vi "Create File.vi"(8 "error in (no error)":errorcluster, 9 "Numeric":dbl, 10 "Folder Name Prefix":string) -> (0 "error out":errorcluster, 2 "refnum out":refnum<file>)   [LabVIEW 2015]
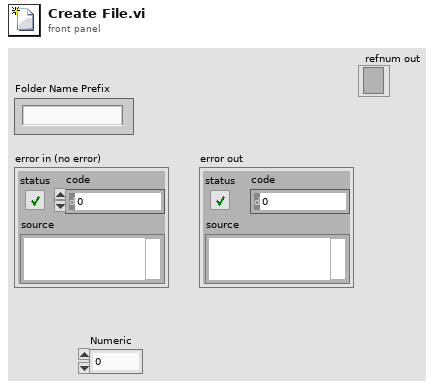
[diagram p1: front panel]
types:
  T1 = enum16{"open", "replace", "create", "open or create", "replace or create", "replace or create with confirmation"}
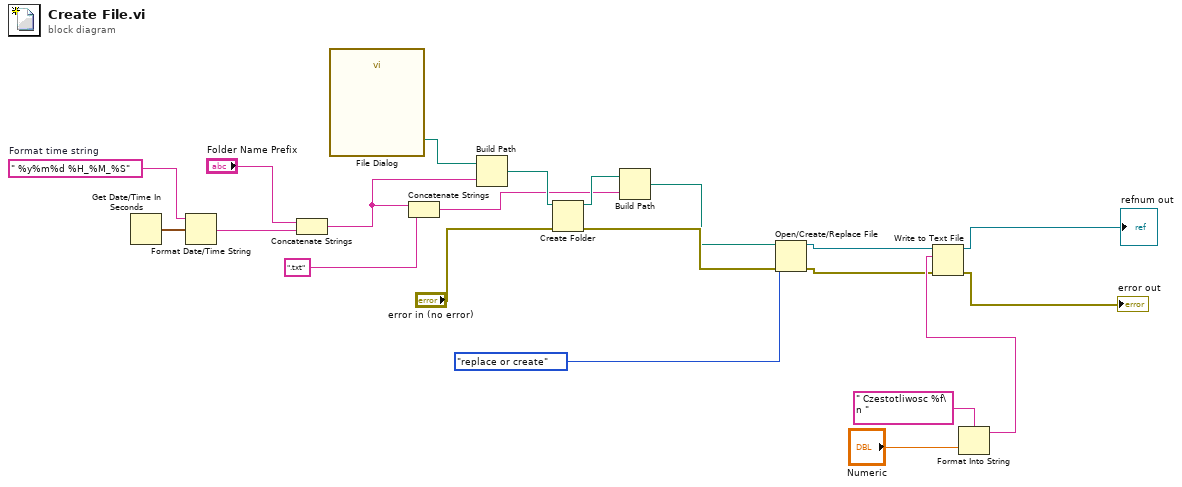
[diagram p0: block diagram]
diagram:
  w18 = " %y%m%d %H_%M_%S"  # Format time string
  n1 = Get Date/Time In Seconds() -> (seconds since 1Jan1904=w16:timestamp)
  n2 = Format Date/Time String(time format string (%c)=w18, seconds (now)=w16) -> (date/time string=w19:string)  [unwired: 1 in]
  n3 = Concatenate Strings("Folder Name Prefix", w19) -> (w10:string)
  n4 = call "File Dialog"() -> ("selected path"=w20:path)  [unwired: 12 in, 3 out]
  n5 = Concatenate Strings(w10, ".txt" ("string")) -> (w8:string)
  n6 = Build Path(base path=w20, name or relative path=w10) -> (appended path=w15:path)
  n7 = Create Folder(path (use dialog)=w15, error in="error in (no error)") -> (created path=w12:path, error out=w13:errorcluster)  [unwired: 1 in, 1 out]
  n8 = Build Path(base path=w12, name or relative path=w8) -> (appended path=w11:path)
  n9 = Open/Create/Replace File(file path (use dialog)=w11, error in=w13, operation (0:open)=T1."replace or create") -> (refnum out=w4:refnum<file>, error out=w1:errorcluster)  [unwired: 3 in, 1 out]
  n10 = Format Into String(format string=" Czestotliwosc %f\n ", "Numeric") -> (resulting string=w5:string)  [unwired: 2 in, 1 out]
  n11 = Write to Text File(file (use dialog)=w4, text=w5, error in=w1) -> (refnum out=→"refnum out":refnum<file>, error out=→"error out":errorcluster)  [unwired: 1 in, 1 out]
